vi "Vобр.vi"(1 "Длина, мм.":dbl=8.0 min=8.0 max=150.0, 2 "Диаметр. мм.":dbl=8.0 min=8.0 max=100.0) -> (0 "Объем образца см3":dbl)   [LabVIEW 2018]
panel:
  out "Объем образца см3 222":dbl
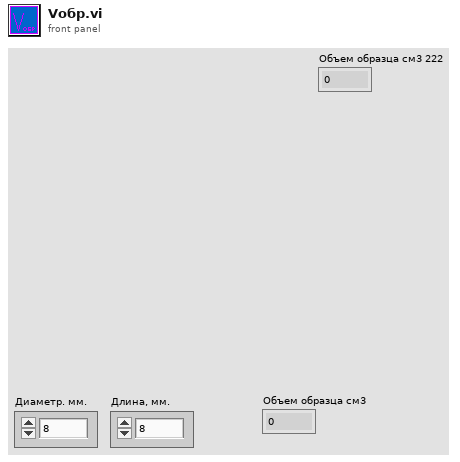
[diagram p1: front panel]
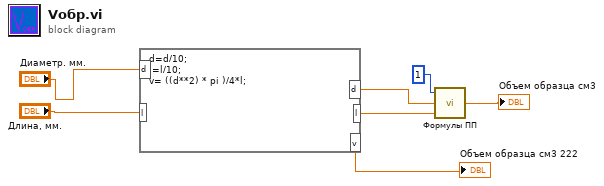
[diagram p0: block diagram]
diagram:
  n1 = formula code="d=d/10;\nl=l/10;\nv= ((d**2) * pi )/4*l;"("d"="Диаметр. мм.", "l"="Длина, мм.") -> ("v"=→"Объем образца см3 222":dbl, "l"=w3:dbl, "d"=w2:dbl)
  n2 = call "Формулы ПП.vi"("PerB"=w3, "PerA"=w2, "mode"=1) -> ("Exid"=→"Объем образца см3":dbl)
